vi "HIOKI PW3390 Conf Frequency.vi"(0 "VISA Resource":refnum<visa-resource-name>, 1 "Set/Query (F: Set)":bool, 2 "CH (1)":i32=1 min=1 max=4, 5 "Freq Source (0: U)":enum16{"U", "I"}(ring), 7 "Lowest Freq (3: 5Hz)":T1(ring)=enum."5Hz", 11 "error in (no error)":errorcluster, 12 "OPC query (T: ON)":bool=TRUE, 13 "Error Out (F: Off)":bool) -> (4 "VISA Resource out":refnum<visa-resource-name>, 6 "Freq Source out":enum16{"U", "I"}(ring), 8 "Lowest Freq out":T1(ring)=enum."5Hz", 15 "error out":errorcluster)   [LabVIEW 2009]
doc: "Set/Query\n Set: Send the setting commands for the device.\n Query: Query the setting of the device.\n\nFreq Source\n Sets the frequency measurement source of the specified channel.\n\nLowest Freq\n Sets the measurement lowest frequency."
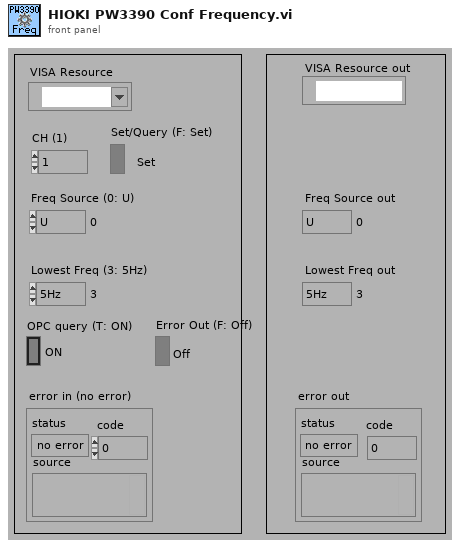
[diagram p1: front panel]
types:
  T1 = enum16{"0.5Hz", "1Hz", "2Hz", "5Hz", "10Hz", "20Hz"}
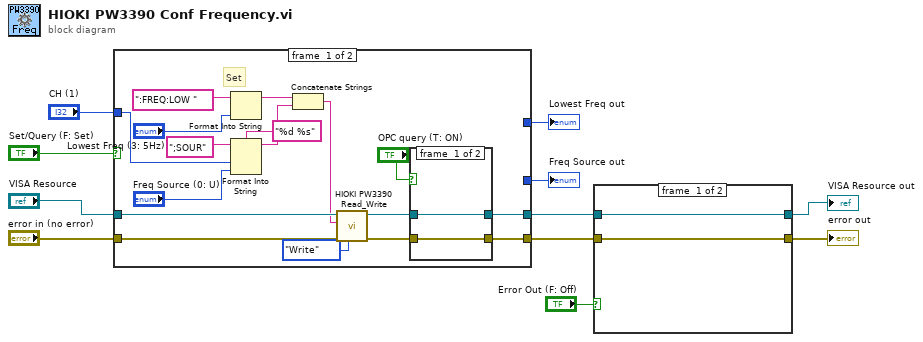
[diagram p0: block diagram]
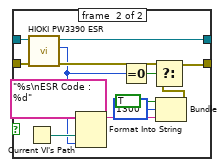
[diagram p2: hidden frame]
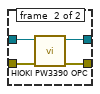
[diagram p3: hidden frame]
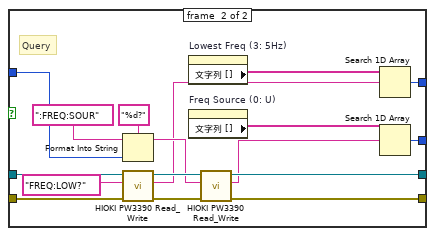
[diagram p4: hidden frame]
diagram:
  n1 = case shown="FALSE" "Set/Query (F: Set)" {
    tunnel: "error in (no error)" -> [w27 w45]
    tunnel: [w12 w49] -> w8
    tunnel: "VISA Resource" -> [w28 w46]
    tunnel: [w13 w48] -> w7
    tunnel: [_ w37] -> w5
    tunnel: [_ w36] -> w4
    tunnel: "CH (1)" -> [w17 w35]
    frame #0 {
      # "Set"
      n2 = Format Into String(initial string=":FREQ:LOW ", "Lowest Freq (3: 5Hz)") -> (resulting string=w22:string)  [unwired: 2 in, 1 out]
      n3 = Format Into String(format string="%d %s", initial string=";SOUR", w17, "Freq Source (0: U)") -> (resulting string=w23:string)  [unwired: 1 in, 1 out]
      n4 = Concatenate Strings(w22, w23) -> (w21:string)
      n5 = call <instrlib>:"HIOKI PW3390 Read_Write.vi"("Read/Write"=enum16{"Read", "Write"}."Write", "error in (no error)"=w27, "data in"=w21, "VISA Resource"=w28) -> ("error out"=w14:errorcluster, "VISA Resource out"=w15:refnum<visa-resource-name>)  [unwired: 5 in, 1 out]
      n6 = case shown="TRUE" "OPC query (T: ON)" {
        tunnel: [w30 w34] -> w13
        tunnel: [w29 w33] -> w12
        tunnel: w15 -> [w30 w32]
        tunnel: w14 -> [w29 w31]
        frame #0 {
        }
        frame #1 {
          n7 = call <instrlib>:"HIOKI PW3390 OPC.vi"("error in (no error)"=w31, "VISA Resource"=w32) -> ("error out"=w33:errorcluster, "VISA Resource out"=w34:refnum<visa-resource-name>)  [unwired: 7 in, 1 out]
        }
      }
    }
    frame #1 {
      # "Query"
      n8 = Format Into String(format string="%d?", initial string=":FREQ:SOUR", w35) -> (resulting string=w42:string)  [unwired: 1 in, 1 out]
      n9 = call <instrlib>:"HIOKI PW3390 Read_Write.vi"("error in (no error)"=w45, "data in"="FREQ:LOW?", "VISA Resource"=w46) -> ("error out"=w51:errorcluster, "data out"=w40:string, "VISA Resource out"=w50:refnum<visa-resource-name>)  [unwired: 6 in]
      n10 = property on="Lowest Freq (3: 5Hz)" class="Enum (strict)"() -> ("文字列 []"=w41:string[])  [unwired: 2 in, 2 out]
      n11 = property on="Freq Source (0: U)" class="Enum (strict)"() -> ("文字列 []"=w39:string[])  [unwired: 2 in, 2 out]
      n12 = call <instrlib>:"HIOKI PW3390 Read_Write.vi"("error in (no error)"=w51, "data in"=w42, "VISA Resource"=w50) -> ("error out"=w49:errorcluster, "data out"=w38:string, "VISA Resource out"=w48:refnum<visa-resource-name>)  [unwired: 6 in]
      n13 = Search 1D Array(1D array=w41, element=w40) -> (index of element=w36:i32)  [unwired: 1 in]
      n14 = Search 1D Array(1D array=w39, element=w38) -> (index of element=w37:i32)  [unwired: 1 in]
    }
  }
  "Lowest Freq out" <- w4
  "Freq Source out" <- w5
  n15 = case shown="TRUE" "Error Out (F: Off)" {
    tunnel: w7 -> [w53 w66]
    tunnel: w8 -> [w52 w65]
    tunnel: [w52 w55] -> w6
    tunnel: [w53 w64] -> w1
    frame #0 {
    }
    frame #1 {
      n16 = Current VI's Path() -> (path=w62:path)
      n17 = call <instrlib>:"HIOKI PW3390 ESR.vi"("error in (no error)"=w65, "VISA Resource"=w66) -> ("error out"=w56:errorcluster, "Output Value"=w54:u8, "VISA Resource out"=w64:refnum<visa-resource-name>)  [unwired: 6 in, 1 out]
      n18 = Format Into String(format string="%s\nESR Code : %d", w62, w54) -> (resulting string=w58:string)  [unwired: 2 in, 1 out]
      n19 = Equal To 0?(x=w54) -> (x = 0?=w63:bool)
      n20 = Bundle("status"=TRUE, "code"=1300, w58) -> (w57:cluster{"status":bool, "code":i32, string})  [unwired: 1 in]
      n21 = Select(t=w56, s=w63, f=w57) -> (s? t:f=w55:errorcluster)
    }
  }
  "error out" <- w6
  "VISA Resource out" <- w1
